vi "Wench Controller.vi"(6 "stop wenching back":bool, 8 "catapult from shift":T1, 9 "arm button":bool, 10 "LimitSwich":bool, 11 "Trigger":bool) -> (0 "catapult to shift":T1, 1 "Ready To Fire":bool, 2 "Cylinder output":bool, 3 "Motor output":dbl)   [LabVIEW 2013]
uses:
  catapult shift.ctl
  cataplut states.ctl
  <vilib>/Rock Robotics/WPI/Solenoid/WPI_SolenoidValue.ctl
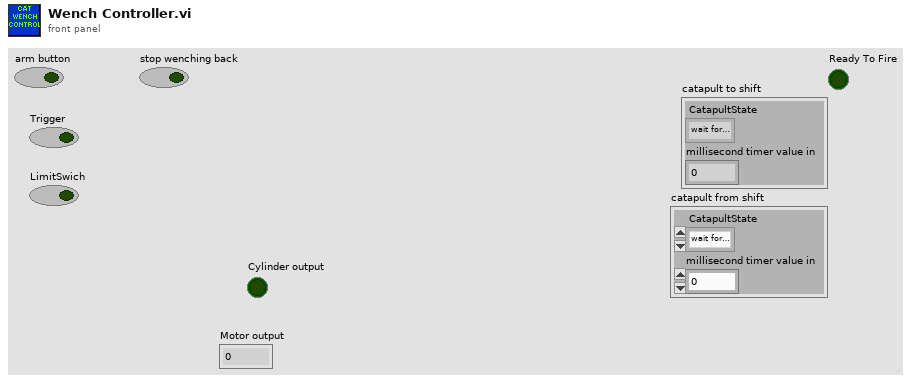
[diagram p1: front panel]
types:
  T1 = typedef "catapult shift.ctl" = cluster{" CatapultState":T2, "millisecond timer value in":u32}
  T2 = typedef "cataplut states.ctl" = enum16{"wait for trigger", "firing", "wait for coming back", "wench back"}
  T3 = typedef "WPI_SolenoidValue.ctl" = enum16{"Off", "On", "Forward", "Reverse"}
  T4 = cluster{"Enum 2":T2, "millisecond timer value in":u32}
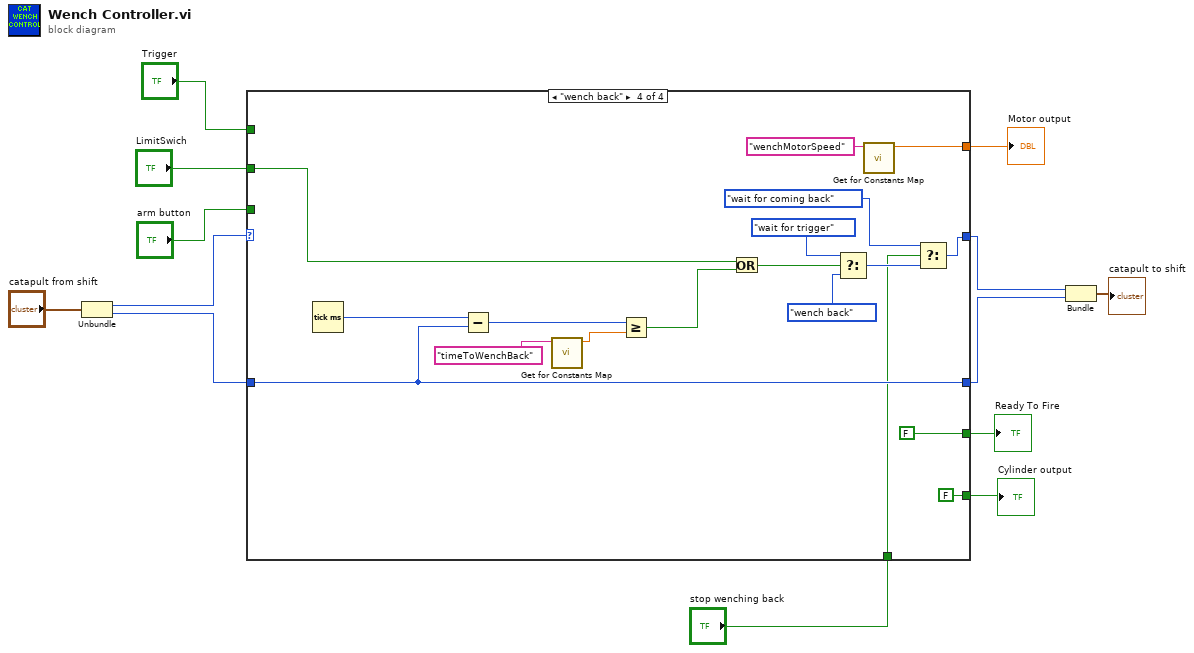
[diagram p0: block diagram]
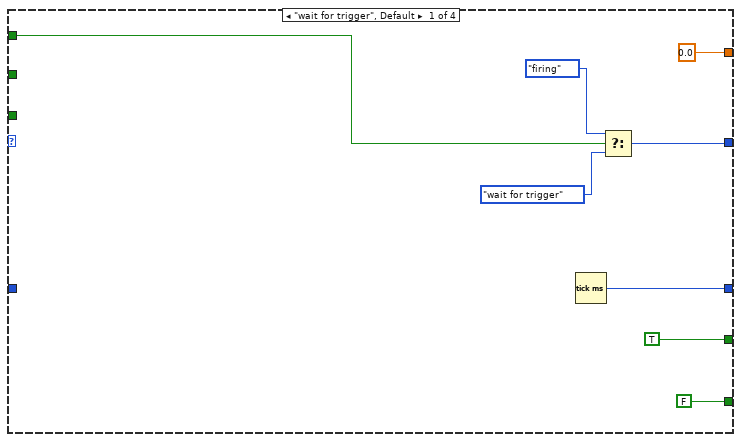
[diagram p2: hidden frame]
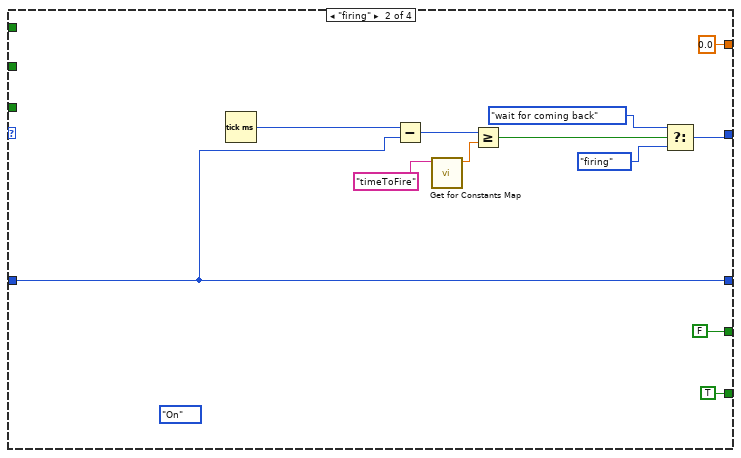
[diagram p3: hidden frame]
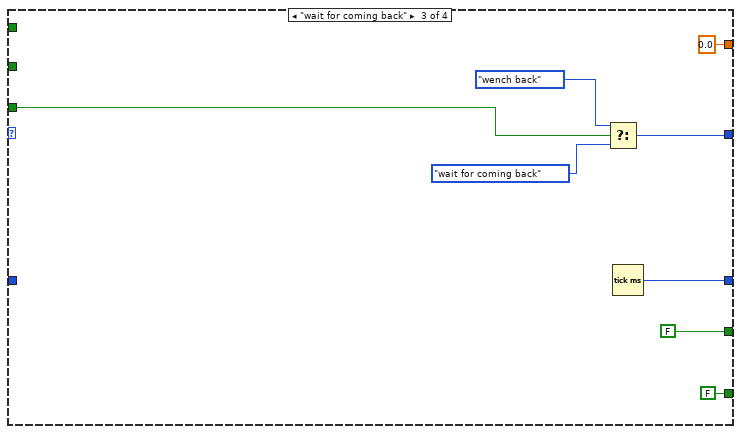
[diagram p4: hidden frame]
diagram:
  n1 = Unbundle("catapult from shift") -> ("CatapultState"=w4:T2, "millisecond timer value in"=w5:u32)
  n2 = case shown="\"wench back\"" w4 {
    tunnel: "Trigger" -> [w21 _ _ _]
    tunnel: [w19 w33 w36 w44] -> w9
    tunnel: [w17 w23 w35 w56] -> w8
    tunnel: w5 -> [_ w23 _ w56]
    tunnel: "LimitSwich" -> [_ _ _ w54]
    tunnel: [0.0 ("Motor output") 0.0 ("Motor output") 0.0 ("Motor output") w46] -> w11
    tunnel: [FALSE ("Cylinder output") TRUE ("Cylinder output") FALSE ("Cylinder output") FALSE ("Cylinder output")] -> w10
    tunnel: "arm button" -> [_ _ w37 _]
    tunnel: [TRUE ("Ready To Fire") FALSE ("Ready To Fire") FALSE ("Ready To Fire") FALSE ("Ready To Fire")] -> w2
    tunnel: "stop wenching back" -> [_ _ _ w42]
    frame "wait for trigger", Default {
      n3 = Tick Count (ms)() -> (millisecond timer value=w17:u32)
      n4 = Select(t=cataplut_states."firing" ("Enum 2"), s=w21, f=cataplut_states."wait for trigger" ("Enum 2")) -> (s? t:f=w19:T2)
    }
    frame "firing" {
      (unwired) WPI_SolenoidValue."On" ("Value")
      n5 = Tick Count (ms)() -> (millisecond timer value=w29:u32)
      n6 = Subtract(x=w29, y=w23) -> (x-y=w30:u32)
      n7 = call "Get for Constants Map.vi"("Constant Name"="timeToFire") -> ("Value"=w27:dbl)  [unwired: 8 in, 2 out]
      n8 = Greater Or Equal?(x=w30, y=w27) -> (x >= y?=w28:bool)
      n9 = Select(t=cataplut_states."wait for coming back" ("Enum 2"), s=w28, f=cataplut_states."firing" ("Enum 2")) -> (s? t:f=w33:T2)
    }
    frame "wait for coming back" {
      n10 = Select(t=cataplut_states."wench back" ("Enum 2"), s=w37, f=cataplut_states."wait for coming back" ("Enum 2")) -> (s? t:f=w36:T2)
      n11 = Tick Count (ms)() -> (millisecond timer value=w35:u32)
    }
    frame "wench back" {
      n12 = Tick Count (ms)() -> (millisecond timer value=w57:u32)
      n13 = Subtract(x=w57, y=w56) -> (x-y=w55:u32)
      n14 = call "Get for Constants Map.vi"("Constant Name"="timeToWenchBack") -> ("Value"=w51:dbl)  [unwired: 8 in, 2 out]
      n15 = Greater Or Equal?(x=w55, y=w51) -> (x >= y?=w53:bool)
      n16 = Or(x=w54, y=w53) -> (x .or. y?=w52:bool)
      n17 = Select(t=cataplut_states."wait for trigger" ("Enum 2"), s=w52, f=cataplut_states."wench back" ("Enum 2")) -> (s? t:f=w45:T2)
      n18 = call "Get for Constants Map.vi"("Constant Name"="wenchMotorSpeed") -> ("Value"=w46:dbl)  [unwired: 8 in, 2 out]
      n19 = Select(t=cataplut_states."wait for coming back" ("Enum 2"), s=w42, f=w45) -> (s? t:f=w44:T2)
    }
  }
  "Motor output" <- w11
  "Cylinder output" <- w10
  "Ready To Fire" <- w2
  n20 = Bundle("Enum 2"=w9, "millisecond timer value in"=w8) -> (→"catapult to shift":T4)  [unwired: 1 in]
